vi "Set Text.vi"(8 "error in (no error)":errorcluster, 9 "Text":string="Hello world!", 10 "Shapre refnum":refnum<k7>) -> (0 "error out":errorcluster, 2 "Shapre refnum out":refnum<k7>)   [LabVIEW 2020, in "lvpptx.lvlib"]
uses:
  lvpptx.lvlib
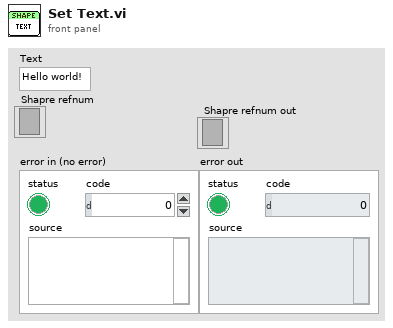
[diagram p1: front panel]
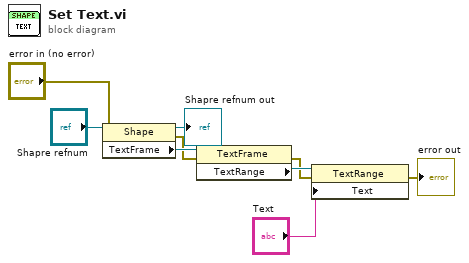
[diagram p0: block diagram]
diagram:
  n1 = property class="Shape"(reference="Shapre refnum", error in="error in (no error)") -> (reference out=→"Shapre refnum out":refnum<k7>, error out=w6:errorcluster, "TextFrame"=w9:refnum<k7>)
  n2 = property class="TextFrame"(reference=w9, error in=w6) -> (error out=w5:errorcluster, "TextRange"=w8:refnum<k7>)  [unwired: 1 out]
  n3 = property class="TextRange"(reference=w8, error in=w5, "Text"="Text") -> (error out=→"error out":errorcluster)  [unwired: 1 out]
